vi "Custom temp ctrl - Setpoint.vi"(8 "Error In":errorcluster, 10 "Setpoint":dbl[unit], 11 "Temp ctrl":T1={"Gain (P)"=0.0, "Reset (I)"=0.0, "Rate (D)"=0.0, "Stabilization rate"=0.0, "Stabilization delta"=0.0, "Type"=enum."Lake Shore 325", "Custom temp ctrl"={"VISA resource name"=""}, "Lakeshore 325"={"VISA name"="", "Loop"=1, "Heater Range"=0, "Heater Resistance"=1, "Sample sensor"=0, "Fast sensor"=0, "Slow sensor"=0}, "Lakeshore 331"={"VISA name"="", "Loop"=1, "Heater Range"=0, "Sample sensor"=0, "Fast sensor"=0, "Slow sensor"=0}, "Lakeshore 332"={"VISA name"="", "Loop"=1, "Heater Range"=0, "Sample sensor"=0, "Fast sensor"=0, "Slow sensor"=0}, "Lakeshore 335"={"VISA name"="", "Loop"=1, "Sample sensor"=0, "Fast sensor"=0, "Slow sensor"=0, "Heater Range"=0, "Output mode"=enum."Off"}, "Lakeshore 336"={"VISA name"="", "Loop"=1, "Output mode"=enum."Off", "Max current"=1.0, "Heater resistance"=1, "Sample sensor"=1, "Slow sensor"=1, "Fast sensor"=1}} {"Lakeshore 336"."Fast sensor" items=["Sensor A", "Sensor B", "Sensor C", "Sensor D"]; "Lakeshore 336"."Slow sensor" items=["Sensor A", "Sensor B", "Sensor C", "Sensor D"]; "Lakeshore 336"."Sample sensor" items=["Sensor A", "Sensor B", "Sensor C", "Sensor D"]; "Lakeshore 336"."Heater resistance" items=["25 Ohm"=1, "50 Ohm"=2]; "Lakeshore 336"."Max current" items=["0.707 A"=0.0, "1 A"=1.0, "1.414 A"=1.414, "2 A"=2.0]; "Lakeshore 336"."Loop" items=["Output 1"=1, "Output 2"=2, "Output 3"=3, "Output 4"=4]; "Lakeshore 335"."Heater Range" items=["Off", "Low (On)", "Medium", "High"]; "Lakeshore 335"."Slow sensor" items=["A", "B"]; "Lakeshore 335"."Fast sensor" items=["A", "B"]; "Lakeshore 335"."Sample sensor" items=["A", "B"]; "Lakeshore 335"."Loop" items=["Loop 1"=1, "Loop 2"=2]; "Lakeshore 332"."Slow sensor" items=["A", "B"]; "Lakeshore 332"."Fast sensor" items=["A", "B"]; "Lakeshore 332"."Sample sensor" items=["A", "B"]; "Lakeshore 332"."Heater Range" items=["Off", "Low (0.5W)", "Med (5W)", "High (50W)"]; "Lakeshore 332"."Loop" items=["Loop 1", "Loop 2"]; "Lakeshore 331"."Slow sensor" items=["A", "B"]; "Lakeshore 331"."Fast sensor" items=["A", "B"]; "Lakeshore 331"."Sample sensor" items=["A", "B"]; "Lakeshore 331"."Heater Range" items=["Off", "Low (0.5W)", "Med (5W)", "High (50W)"]; "Lakeshore 331"."Loop" items=["Loop 1", "Loop 2"]; "Lakeshore 325"."Slow sensor" items=["A", "B"]; "Lakeshore 325"."Fast sensor" items=["A", "B"]; "Lakeshore 325"."Sample sensor" items=["A", "B"]; "Lakeshore 325"."Heater Resistance" items=["25 Ohm"=1, "50 Ohm"=2]; "Lakeshore 325"."Heater Range" items=["Off", "Low (loop 1) or On (loop 2)", "High (loop 1)"]; "Lakeshore 325"."Loop" items=["Loop 1"=1, "Loop 2"=2]}) -> (0 "Error Out":errorcluster)   [LabVIEW 2019]
doc: "This subVI is meant to perform all operations necessary to apply a temperature setpoint to your temperature controller. Setpoint and Temp handle parameters, including your custom settings are made available to you."
uses:
  Type defs/Temp ctrl Type Def.ctl
  Custom temp ctrl settings.ctl
panel:
  # "Place all operations necessary to apply setpoint to your custom temperature controler in this VI"
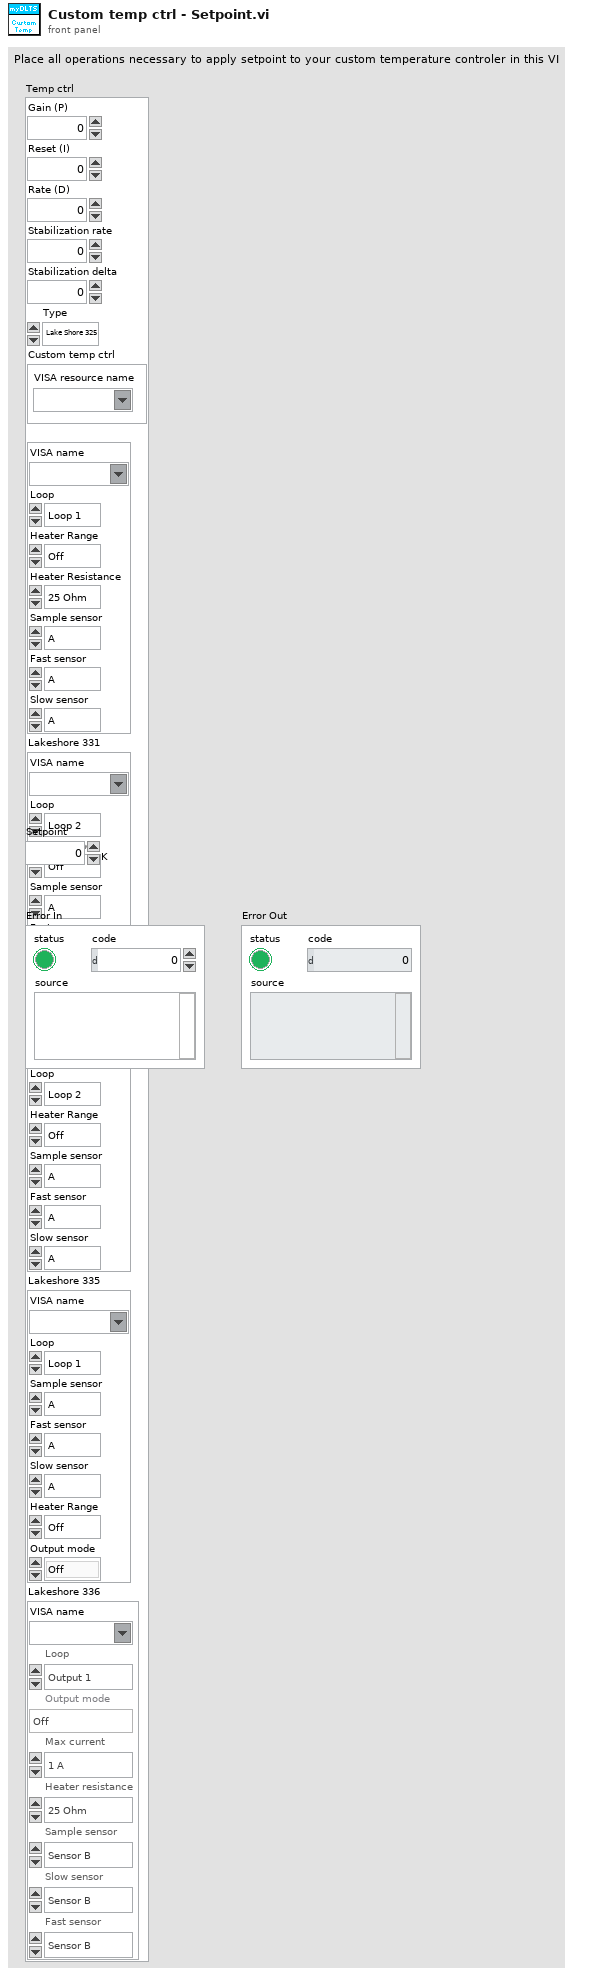
[diagram p1: front panel]
types:
  T1 = typedef "Temp ctrl Type Def.ctl" = cluster{"Gain (P)":dbl, "Reset (I)":dbl, "Rate (D)":dbl, "Stabilization rate":dbl, "Stabilization delta":dbl, "Type":enum16{"Custom", "Lake Shore 325", "Lake Shore 331", "Lake Shore 332", "Lake Shore 335", "Lake Shore 336"}, "Custom temp ctrl":T2, "Lakeshore 325":cluster{"VISA name":refnum<visa-resource-name>, "Loop":u16, "Heater Range":u16, "Heater Resistance":u16, "Sample sensor":u16, "Fast sensor":u16, "Slow sensor":u16}, "Lakeshore 331":cluster{"VISA name":refnum<visa-resource-name>, "Loop":u16, "Heater Range":u16, "Sample sensor":u16, "Fast sensor":u16, "Slow sensor":u16}, "Lakeshore 332":cluster{"VISA name":refnum<visa-resource-name>, "Loop":u16, "Heater Range":u16, "Sample sensor":u16, "Fast sensor":u16, "Slow sensor":u16}, "Lakeshore 335":cluster{"VISA name":refnum<visa-resource-name>, "Loop":u16, "Sample sensor":u16, "Fast sensor":u16, "Slow sensor":u16, "Heater Range":u16, "Output mode":enum16{"Off", "Closed Loop PID", "Zone", "Open Loop", "Monitor Out", "Warmup Supply"}}, "Lakeshore 336":cluster{"VISA name":refnum<visa-resource-name>, "Loop":u16, "Output mode":enum16{"Off", "Closed Loop PID", "Zone", "Open Loop"}, "Max current":dbl, "Heater resistance":u16, "Sample sensor":u16, "Slow sensor":u16, "Fast sensor":u16}}
  T2 = typedef "Custom temp ctrl settings.ctl" = cluster{"VISA resource name":refnum<visa-resource-name>}
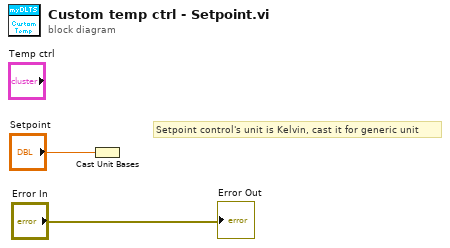
[diagram p0: block diagram]
diagram:
  # "Setpoint control's unit is Kelvin, cast it for generic unit"
  n1 = Cast Unit Bases(0:"Setpoint") -> ()  [unwired: 1 in, 1 out]
  "Error Out" <- "Error In"
